vi "getItem.vi"(8 "error in (no error)":errorcluster, 10 "LocalId in":string, 11 "IFolder in":refnum<class "IFolder.lvclass">) -> (0 "error out":errorcluster, 1 "LocalId out":string, 2 "Components out":refnum<class "IComponent.lvclass">, 3 "IFolder out":refnum<class "IFolder.lvclass">)   [LabVIEW 2022 SP3, in "openDAQ.lvlib" / "IBaseObject.lvlib" / "IPropertyObject.lvlib" / "IComponent.lvlib" / "IFolder.lvlib" / "IFolder.lvclass"]
uses:
  <instrlib>/openDAQ/Public/Classes/IFolder/IFolder.lvclass
  <instrlib>/openDAQ/Public/Classes/IFolder/IFolder.lvclass/IFolder.ctl
  <instrlib>/openDAQ/Public/Classes/IComponent/IComponent.lvclass
  <instrlib>/openDAQ/Binaries/Windows/x86/copendaq32.dll
  <instrlib>/openDAQ/Public/Classes/daqCoreTypes/IString/IString.lvclass
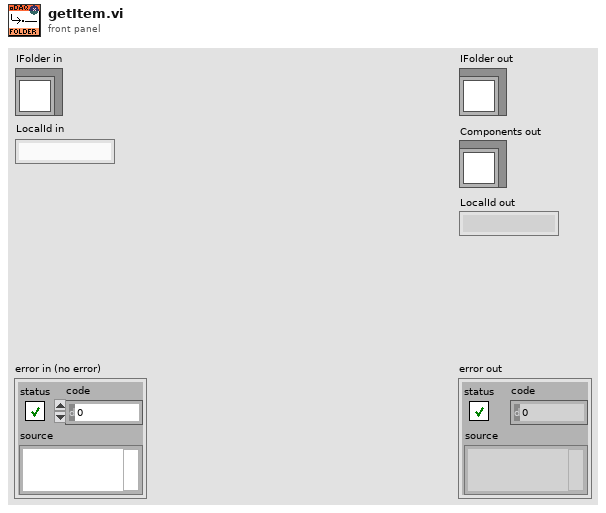
[diagram p1: front panel]
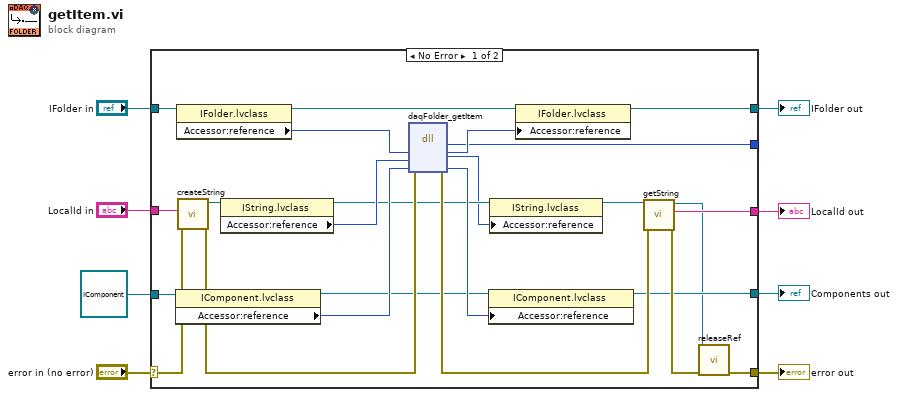
[diagram p0: block diagram]
diagram:
  n1 = case shown="No Error" "error in (no error)" {
    selector: "error in (no error)" -> [w17 w35]
    tunnel: [w10 w35] -> w7
    tunnel: [w21 w34] -> w5
    tunnel: "IFolder in" -> [w26 w34]
    tunnel: refnum<class "IComponent.lvclass"> refnum ("openDAQ.lvlib:IBaseObject.lvlib:IPropertyObject.lvlib:IComponent.lvlib:IComponent.lvclass") -> [w25 _]
    tunnel: [w11 _] -> w3
    tunnel: [w19 _] -> _
    tunnel: "LocalId in" -> [w18 w33]
    tunnel: [w30 w33] -> w1
    frame No Error {
      n2 = property class="IComponent.lvclass"(reference=w25) -> (reference out=w20:refnum<class "IComponent.lvclass">, "Accessor:reference"=w28:i64)  [unwired: 1 in, 1 out]
      n3 = property class="IFolder.lvclass"(reference=w26) -> (reference out=w22:refnum<class "IFolder.lvclass">, "Accessor:reference"=w24:i64)  [unwired: 1 in, 1 out]
      n4 = call <instrlib>:"createString.vi"("error in (no error)"=w17, "String"=w18) -> ("error out"=w29:errorcluster, "IString out"=w16:refnum<class "IString.lvclass">)  [unwired: 8 in]
      n5 = property class="IString.lvclass"(reference=w16) -> (reference out=w14:refnum<class "IString.lvclass">, "Accessor:reference"=w15:i64)  [unwired: 1 in, 1 out]
      n6 = dll-call lib="C:/Program Files (x86)/National Instruments/LabVIEW 2022/instr.lib/openDAQ/Binaries/Windows/x86/copendaq*.*" fn="daqFolder_getItem"(error in=w29, "folder"=w24, "localId"=w15, "item"=w28) -> (error out=w31:errorcluster, "return type"=w19:u32, "folder"=w23:i64, "localId"=w13:i64, "item"=w27:i64)  [unwired: 2 in, 1 out]
      n7 = property class="IComponent.lvclass"(reference=w20, "Accessor:reference"=w27) -> (reference out=w11:refnum<class "IComponent.lvclass">)  [unwired: 1 in, 1 out]
      n8 = property class="IString.lvclass"(reference=w14, "Accessor:reference"=w13) -> (reference out=w12:refnum<class "IString.lvclass">)  [unwired: 1 in, 1 out]
      n9 = property class="IFolder.lvclass"(reference=w22, "Accessor:reference"=w23) -> (reference out=w21:refnum<class "IFolder.lvclass">)  [unwired: 1 in, 1 out]
      n10 = call <instrlib>:"getString.vi"("error in (no error)"=w31, "IString in"=w12) -> ("error out"=w32:errorcluster, "String out"=w30:string, "IString out"=w9:refnum<class "IString.lvclass">)  [unwired: 7 in]
      n11 = call-dynamic "releaseRef.vi"("error in (no error)"=w32, "IBaseObject in"=w9) -> ("error out"=w10:errorcluster)  [unwired: 9 in]
    }
    frame Error {
    }
  }
  "error out" <- w7
  "IFolder out" <- w5
  "Components out" <- w3
  "LocalId out" <- w1
